vi "NI VeriStand - Close Runtime Confgiuration Ref.vi"(8 "error in":errorcluster, 11 "Runtime Configuration Ref in":refnum<k39>) -> (0 "error out":errorcluster)   [LabVIEW 2027, in "Runtime Configuration File API.lvlib"]
uses:
  Runtime Configuration File API.lvlib
  C:/NetCoreDLL/NationalInstruments.VeriStand.SystemDefinitionAPI.dll
  NetCoreDLL/NationalInstruments.VeriStand.SystemDefinitionAPI.dll
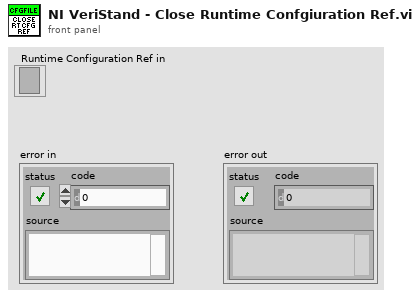
[diagram p1: front panel]
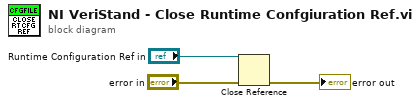
[diagram p0: block diagram]
diagram:
  n1 = Close Reference(reference="Runtime Configuration Ref in", error in (no error)="error in") -> (error out=→"error out":errorcluster)
